vi "MB Registers Read HR.vi"(5 "Data Reference":T1, 8 "error in (no error)":errorcluster, 10 "Length":u16, 11 "Start Address":i16) -> (0 "error out":errorcluster, 1 "Words out":u16[](array[numeric]))   [LabVIEW 2019, in "NI_modbus_upd.lvlib"]
uses:
  Ctl/Data Reference.ctl
  NI_modbus_upd.lvlib
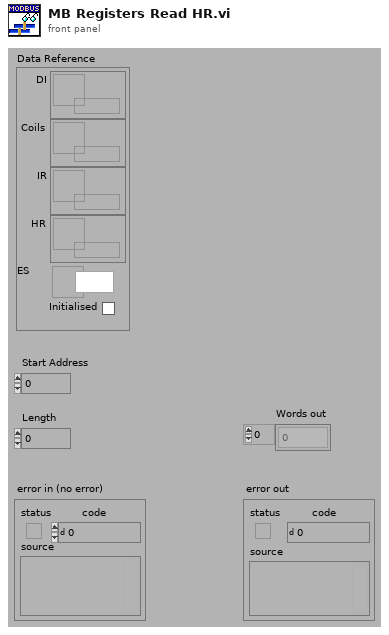
[diagram p1: front panel]
types:
  T1 = typedef "NI_modbus_upd.lvlib/Data Reference.ctl" = cluster{"DI":refnum<data-value>, "Coils":refnum<data-value>, "IR":refnum<data-value>, "HR":refnum<data-value>, "ES":refnum<data-value>, "Initialised":bool}
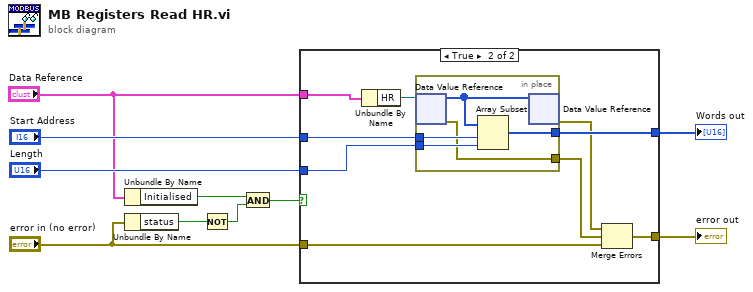
[diagram p0: block diagram]
diagram:
  n1 = Unbundle By Name("Data Reference") -> ("Initialised"=w3:bool)
  n2 = Unbundle By Name("error in (no error)") -> ("status"=w5:bool)
  n3 = Not(x=w5) -> (.not. x?=w4:bool)
  n4 = And(x=w3, y=w4) -> (x .and. y?=w6:bool)
  n5 = case shown="True" w6 {
    tunnel: [w11 w15] -> w10
    tunnel: [_ w20] -> w9
    tunnel: "Length" -> [_ w19]
    tunnel: "Start Address" -> [_ w18]
    tunnel: "Data Reference" -> [_ w17]
    tunnel: "error in (no error)" -> [w11 w16]
    frame False {
    }
    frame True {
      n6 = Unbundle By Name(w17) -> ("HR"=w12:refnum<data-value>)
      n7 = in-place {
        in-place-border: w18 -> [w25]
        in-place-border: w19 -> [w24]
        in-place-border: [w22] -> w20
        in-place-border: [w21] -> w13
        n8 = in-place-dvr #1(w12) -> (w23:u16[], w21:errorcluster)
        n9 = Array Subset(array=w23, index=w25, length=w24) -> (w22:u16[])
        n10 = in-place-dvr #1(w23) -> (w14:errorcluster)  [unwired: 1 out]
      }
      n11 = Merge Errors(w14, w13, w16) -> (w15:errorcluster)
    }
  }
  "error out" <- w10
  "Words out" <- w9
